vi "FestoCPX.Station.TowerLed.Set.vi"(8 "error in":errorcluster, 10 "Color (off)":T1, 11 "Blink period [ms] (0)":u32) -> (0 "error out":errorcluster)   [LabVIEW 2016]
uses:
  FestoCPX.Station.TowerLed.Color.ctl
  FestoCPX.DO.Signal.ctl
  FestoCPX.Station.TowerLed.Fglb.Action.ctl
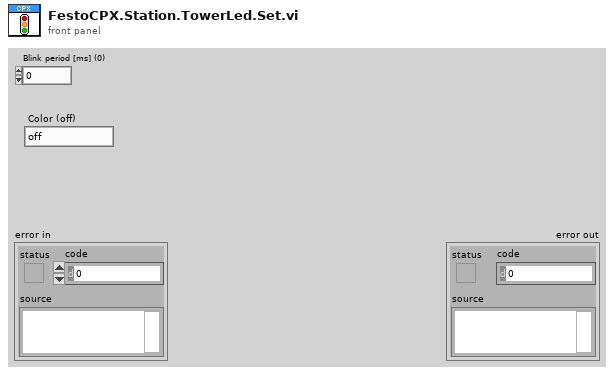
[diagram p1: front panel]
types:
  T1 = typedef "FestoCPX.Station.TowerLed.Color.ctl" = enum16{"off", "red", "orange", "green", "green/orange"}
  T2 = typedef "FestoCPX.Station.TowerLed.Fglb.Action.ctl" = enum16{"init", "set", "get"}
  T3 = typedef "FestoCPX.DO.Signal.ctl" = enum16{"Safety Reset", "Air Main Valve", "Door Lock", "Button LED Start", "Button LED Stop", "Button LED Control", "Traffic LED Red", "Traffic LED Orange", "Traffic LED Green", "Horn", "Laser Interlock", "Laser Trigger", "Laser Fume Extractor", "Product Suction Gripper Slot 1 A", "Product Suction Gripper Slot 1 B", "Product Suction Gripper Slot 2 A", "Product Suction Gripper Slot 2 B", "Product Suction Gripper Slot 3 A", "Product Suction Gripper Slot 3 B", "Product Suction Gripper Slot 4 A", "Product Suction Gripper Slot 4 B", "Product Suction Gripper Final A", "Product Suction Gripper Final B", "Lamp", "Q1 Product Move Work", "Q1 Product Move Home", "Q2 Table Turn Work", "Q2 Table Turn Home", "Q3 Product Lift A", "Q3 Product Lift B", "Q4 Product Arm OK", "Q4 Product Arm NOK", "Q5 Product Arm Work", "Q6 Product BlowOut A", "Q6 Product BlowOut B"}
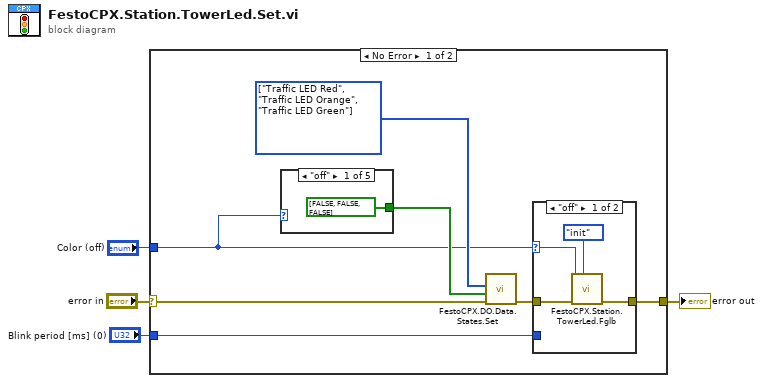
[diagram p0: block diagram]
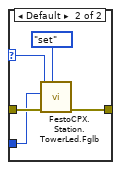
[diagram p2: hidden frame]
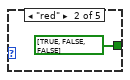
[diagram p3: hidden frame]
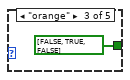
[diagram p4: hidden frame]
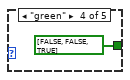
[diagram p5: hidden frame]
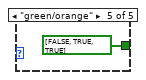
[diagram p6: hidden frame]
diagram:
  n1 = case shown="No Error" "error in" {
    selector: "error in" -> [w11 w26]
    tunnel: [w7 w26] -> w4
    tunnel: "Color (off)" -> [w6 _]
    tunnel: "Blink period [ms] (0)" -> [w5 _]
    frame No Error {
      w9 = T3[] [enum."Traffic LED Red", enum."Traffic LED Orange", enum."Traffic LED Green"] items=["Safety Reset", "Air Main Valve", "Door Lock", "Button LED Start", "Button LED Stop", "Button LED Control", "Traffic LED Red", "Traffic LED Orange", "Traffic LED Green", "Horn", "Laser Interlock", "Laser Trigger", "Laser Fume Extractor", "Product Suction Gripper Slot 1 A", "Product Suction Gripper Slot 1 B", "Product Suction Gripper Slot 2 A", "Product Suction Gripper Slot 2 B", "Product Suction Gripper Slot 3 A", "Product Suction Gripper Slot 3 B", "Product Suction Gripper Slot 4 A", "Product Suction Gripper Slot 4 B", "Product Suction Gripper Final A", "Product Suction Gripper Final B", "Lamp", "Q1 Product Move Work", "Q1 Product Move Home", "Q2 Table Turn Work", "Q2 Table Turn Home", "Q3 Product Lift A", "Q3 Product Lift B", "Q4 Product Arm OK", "Q4 Product Arm NOK", "Q5 Product Arm Work", "Q6 Product BlowOut A", "Q6 Product BlowOut B"] ("CPX.DO")
      n2 = case shown="\"off\"" w6 {
        tunnel: [bool[] [FALSE, FALSE, FALSE] bool[] [TRUE, FALSE, FALSE] bool[] [FALSE, TRUE, FALSE] bool[] [FALSE, FALSE, TRUE] bool[] [FALSE, TRUE, TRUE]] -> w10
        frame "off" {
        }
        frame "red" {
        }
        frame "orange" {
        }
        frame "green" {
        }
        frame "green/orange" {
        }
      }
      n3 = call "FestoCPX.DO.Data.States.Set.vi"("error in (no error)"=w11, "State"=w10, "CPX.DO"=w9) -> ("error out"=w8:errorcluster)  [unwired: 8 in]
      n4 = case shown="\"off\"" w6 {
        selector: w6 -> [w12 w17]
        tunnel: w8 -> [w15 w20]
        tunnel: [w14 w19] -> w7
        tunnel: w5 -> [_ w16]
        frame "off" {
          n5 = call "FestoCPX.Station.TowerLed.Fglb.vi"("Action (get)"=FestoCPX.Station.TowerLed.Fglb.Action."init", "error in"=w15, "Color"=w12) -> ("error out"=w14:errorcluster)  [unwired: 6 in, 2 out]
        }
        frame Default {
          n6 = call "FestoCPX.Station.TowerLed.Fglb.vi"("Action (get)"=FestoCPX.Station.TowerLed.Fglb.Action."set", "error in"=w20, "Blink period [ms]"=w16, "Color"=w17) -> ("error out"=w19:errorcluster)  [unwired: 5 in, 2 out]
        }
      }
    }
    frame Error {
    }
  }
  "error out" <- w4
